vi "Rate-Calc.vi"(8 "Pass Through Time":dbl, 11 "Distance":dbl) -> (3 "Rate  /Sec":dbl)   [LabVIEW 2019]
uses:
  <vilib>/Rock Robotics/WPI/ThirdParty/JAS_Junk/TrajLib/Trajectory_Library.lvlib
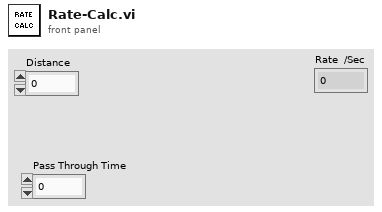
[diagram p1: front panel]
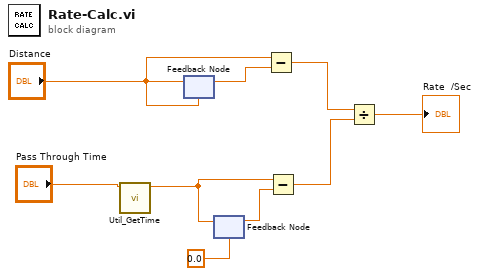
[diagram p0: block diagram]
diagram:
  n1 = call <vilib>:"Util_GetTime.vi"("Pass_Through_Time"="Pass Through Time") -> ("FPGA_Time_Seconds"=w5:dbl)  [unwired: 9 in, 1 out]
  n2 = feedback #1("Distance") -> (w7:dbl)
  n3 = feedback-in #1("Distance") -> ()
  n4 = feedback-in #2(w5) -> ()
  n5 = feedback #2(0.0 ("FPGA_Time_Seconds")) -> (w4:dbl)
  n6 = Subtract(x="Distance", y=w7) -> (x-y=w3:dbl)
  n7 = Subtract(x=w5, y=w4) -> (x-y=w2:dbl)
  n8 = Divide(x=w3, y=w2) -> (x/y=→"Rate  /Sec":dbl)
